vi "form_feedback.vi"(11 "JSON":string="{\"cmd\":\"set_feedback\",\"args\":{\"fb channel\":0, \"fb config\":{\"Setpoint\":1, \"Output limit (low)\":-5, \"Output limit (high)\":10, \"P gain\":1e-3, \"I gain\":1e-3, \"Reset\":true, \"Hold\":false, \"Negative\":true, \"Input channel\":0, \"Output channel\":2, \"wait for fb\":false, \"Error limit (high)\":0.1, \"Error limit (low)\":-0.1}}}") -> ()   [LabVIEW 2020]
doc: "Form template VI.\n\nWhen you want to create a new form, please copy and modify this VI.\nThe form vi should be placed in the host/form directory."
uses:
  fpga/fpga_feedback_config.ctl
  core/host_global_vars.vi
  <vilib>/rvi/interface/RandomDataEmulation/niFpgaReadControlTemplate.vi
  <vilib>/rvi/interface/RandomDataEmulation/niFpgaWriteControlTemplate.vi
  <vilib>/rvi/interface/nirviReadWriteControl/nirviReadWriteControl.xnode
  fpga/fpga_main.vi
panel:
  in  "Feedback 1 config":T1
  in  "Feedback 0 config":T1
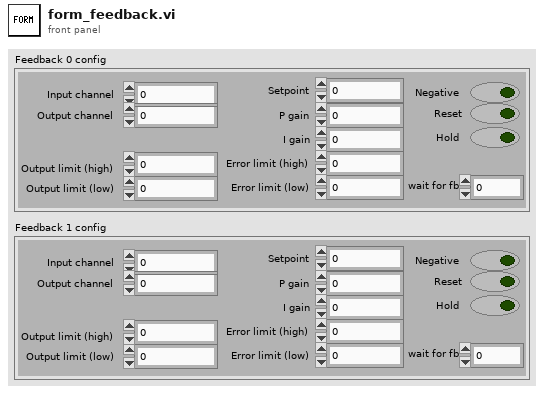
[diagram p1: front panel]
types:
  T1 = typedef "fpga_feedback_config.ctl" = cluster{"Setpoint":sgl, "Output limit (low)":sgl, "Output limit (high)":sgl, "P gain":sgl, "I gain":sgl, "Reset":bool, "Hold":bool, "Negative":bool, "Input channel":i16, "Output channel":i16, "wait for fb":i16, "Error limit (high)":sgl, "Error limit (low)":sgl}
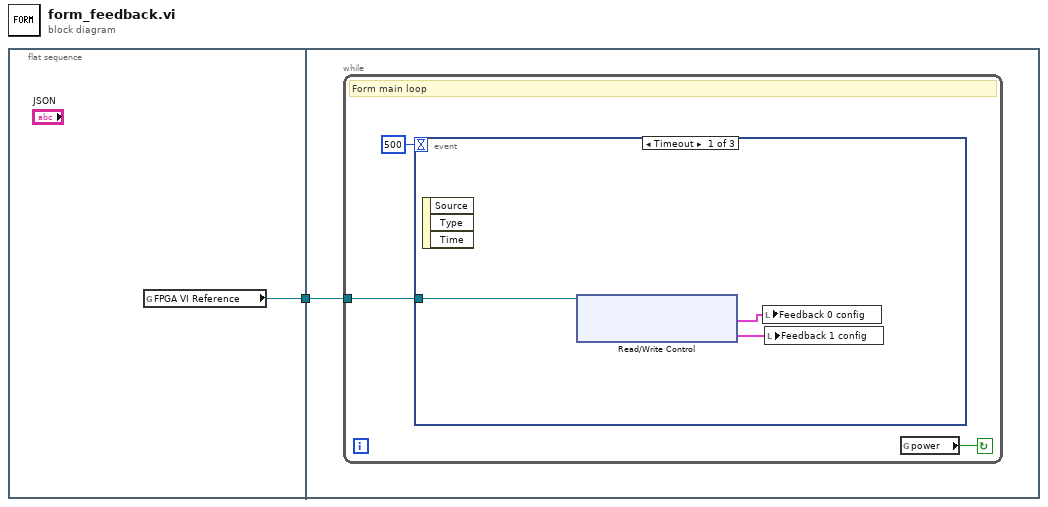
[diagram p0: block diagram]
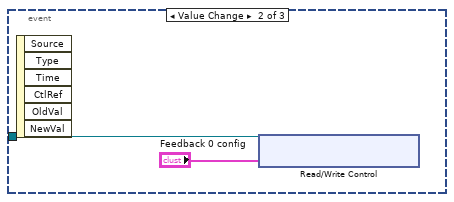
[diagram p2: hidden frame]
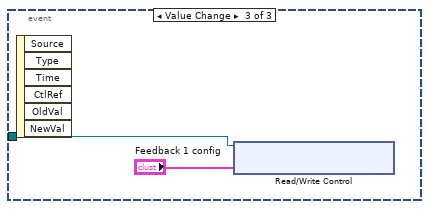
[diagram p3: hidden frame]
diagram:
  n1 = flat-sequence {
    tunnel: [w2] -> w1
    tunnel: w1 -> [w3]
    frame #0 {
      n2 = global read "host_global_vars.vi" "FPGA VI Reference"() -> (w2:refnum<k20>)
    }
    frame #1 {
      n3 = while {
        tunnel: w3 -> [w5]
        stop <- w6 continue-if-true
        # "Form main loop"
        n4 = event shown="[0] Timeout" {
          selector: _ -> [_ _ _]
          dyn-events: _ -> [_ _ _]
          timeout: 500 -> [_ _ _]
          tunnel: w5 -> [w9 w10 w12]
          event Timeout {
            n5 = event-data() -> ()  [unwired: 1 in, 3 out]
            n6 = xnode "Read/Write Control"("FPGA VI Reference In"=w9) -> ("Feedback 0 config"=w8:T1, "Feedback 1 config"=w7:T1)  [unwired: 1 in, 2 out]
            n7 = local write "Feedback 0 config"(w8) -> ()
            n8 = local write "Feedback 1 config"(w7) -> ()
          }
          event Value Change {
            n9 = event-data() -> ()  [unwired: 1 in, 6 out]
            n10 = xnode "Read/Write Control"("FPGA VI Reference In"=w10, "Feedback 0 config"="Feedback 0 config") -> ()  [unwired: 1 in, 2 out]
          }
          event Value Change {
            n11 = event-data() -> ()  [unwired: 1 in, 6 out]
            n12 = xnode "Read/Write Control"("FPGA VI Reference In"=w12, "Feedback 1 config"="Feedback 1 config") -> ()  [unwired: 1 in, 2 out]
          }
        }
        n13 = global read "host_global_vars.vi" "power"() -> (w6:bool)
      }
    }
  }
